vi "Choreo_DifferentialSample_New.vi"(0 "heading":dbl, 1 "velocityL":dbl, 2 "velocityR":dbl, 3 "angularVelocity":dbl, 4 "accelL":dbl, 5 "accelR":dbl, 6 "y":dbl, 7 "accelAngular":dbl, 8 "x":dbl, 9 "forceL":dbl, 10 "timestamp":dbl, 11 "forceR":dbl) -> (14 "ChoreoDifferentialSample":T1={"timestamp"=-999.0, "x"=0.0, "y"=0.0, "heading"=0.0, "velocityL"=0.0, "velocityR"=0.0, "angularVelocity"=0.0, "accelL"=0.0, "accelR"=0.0, "accelAngular"=0.0, "forceL"=0.0, "forceR"=0.0})   [LabVIEW 2019, in "ChoreoLib.lvlib"]
doc: "Constructs a DifferentialSample with the specified parameters.\n\nInputs: \n - timestamp - double - The timestamp of this sample relative to the beginning of the trajectory. \n - x - double - The X position of the sample relative to the blue alliance wall origin in meters. \n - y- double - The Y position of the sample relative to the blue alliance wall origin in meters. \n - heading - double - The heading of the sample in radians, with 0 being in the +X direction. \n - velocityL- double - The velocity of the left side in m/s. \n - velocityR- double - The velocity of the right side in m/s. \n - angularVelocity - double - The chassis angular velocity in rad/s. \n - accelL- double - The acceleration of the left side in m/s². \n - accelR - double - The acceleration of the right side in m/s². \n - accelAngular - double - The chassis angular acceleration in rad/s². \n - forceL - double - The force of the left side in Newtons. \n - forceR - double - The force of the right side in Newtons. \n\nOutputs:\n - ChoreoDifferentialSample - cluster - Cluster containing sample data"
uses:
  ChoreoLib.lvlib
  TypeDef/ChoreoDifferentialSample.ctl
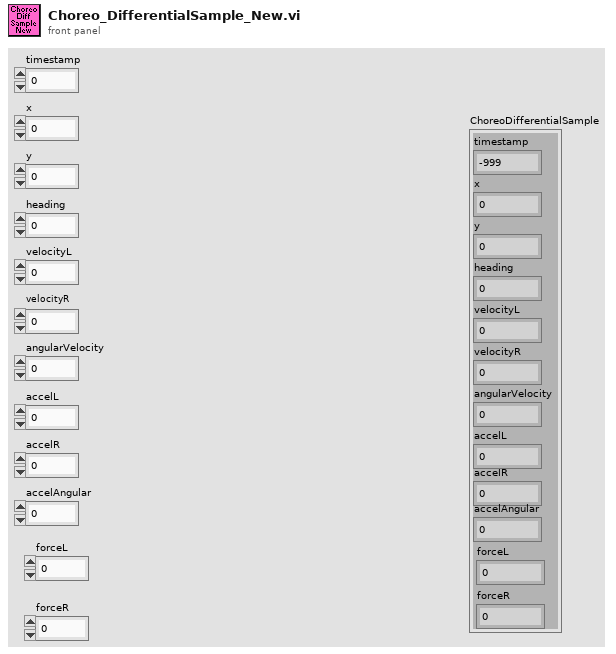
[diagram p1: front panel]
types:
  T1 = typedef "ChoreoLib.lvlib/ChoreoDifferentialSample.ctl" = cluster{"timestamp":dbl, "x":dbl, "y":dbl, "heading":dbl, "velocityL":dbl, "velocityR":dbl, "angularVelocity":dbl, "accelL":dbl, "accelR":dbl, "accelAngular":dbl, "forceL":dbl, "forceR":dbl}
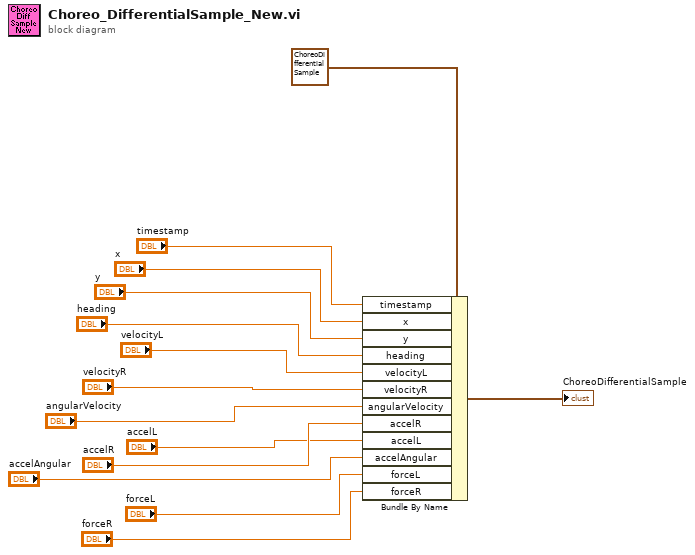
[diagram p0: block diagram]
diagram:
  n1 = Bundle By Name(cluster=T1 {"timestamp"=-999.0, "x"=0.0, "y"=0.0, "heading"=0.0, "velocityL"=0.0, "velocityR"=0.0, "angularVelocity"=0.0, "accelL"=0.0, "accelR"=0.0, "accelAngular"=0.0, "forceL"=0.0, "forceR"=0.0} ("ChoreoSwerveSample"), "timestamp"="timestamp", "x"="x", "y"="y", "heading"="heading", "velocityL"="velocityL", "velocityR"="velocityR", "angularVelocity"="angularVelocity", "accelR"="accelR", "accelL"="accelL", "accelAngular"="accelAngular", "forceL"="forceL", "forceR"="forceR") -> (→"ChoreoDifferentialSample":T1)
